vi "rename.vi"() -> (0 "result string":string)   [LabVIEW 2019]
panel:
  out "after substring":string
  out "time string":string
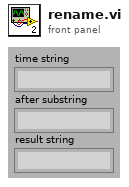
[diagram p1: front panel]
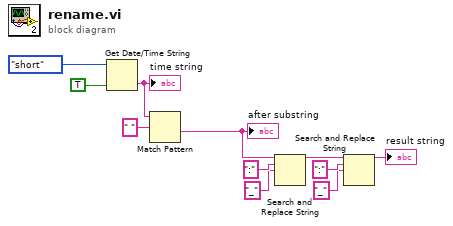
[diagram p0: block diagram]
diagram:
  n1 = Get Date/Time String(date format (0)=enum16{"short", "long", "abbreviated"}."short", want seconds? (F)=TRUE) -> (time string=w9:string)  [unwired: 2 out]
  "time string" <- w9
  n2 = Match Pattern(string=w9, regular expression=" ") -> (after substring=w7:string)  [unwired: 4 out]
  "after substring" <- w7
  n3 = Search and Replace String(input string=w7, search string=":", replace string="_" ("replace string (\"\")")) -> (result string=w4:string)  [unwired: 1 in, 7 out]
  n4 = Search and Replace String(input string=w4, search string=":", replace string="_" ("replace string (\"\")")) -> (result string=→"result string":string)  [unwired: 1 in, 7 out]
